vi "v3.21.v.vi"() -> ()   [LabVIEW 2018]
uses:
  <vilib>/DAQmx/read.llb/DAQmx Read (Analog 1D DBL NChan 1Samp).vi
  <extravilib>/ChannelInstances/High Speed Stream-c(a[.](c(dbl,dbl,dbl,dbl)),stamp,a[.](dbl),c(dbl,dbl,dbl,dbl,dbl,dbl,dbl))/_Read For Replicate.vi
  <extravilib>/ChannelInstances/High Speed Stream-c(a[.](c(dbl,dbl,dbl,dbl)),stamp,a[.](dbl),c(dbl,dbl,dbl,dbl,dbl,dbl,dbl))/Instantiate.vi
  <extravilib>/ChannelInstances/High Speed Stream-c(a[.](c(dbl,dbl,dbl,dbl)),stamp,a[.](dbl),c(dbl,dbl,dbl,dbl,dbl,dbl,dbl))/)Channel.vi
  <extravilib>/ChannelInstances/High Speed Stream-c(a[.](c(dbl,dbl,dbl,dbl)),stamp,a[.](dbl),c(dbl,dbl,dbl,dbl,dbl,dbl,dbl))/Abort Signal/Init Signal.vi
  <vilib>/Utility/file.llb/Write Delimited Spreadsheet (string).vi
  <vilib>/DAQmx/create/channels.llb/DAQmx Create Channel (AI-Temperature-Thermocouple).vi
  <vilib>/DAQmx/configure/timing.llb/DAQmx Timing (Sample Clock).vi
  <vilib>/DAQmx/miscellaneous.llb/DAQmx Fill In Error Info.vi
  <extravilib>/ChannelInstances/High Speed Stream-c(a[.](c(dbl,dbl,dbl,dbl)),stamp,a[.](dbl),c(dbl,dbl,dbl,dbl,dbl,dbl,dbl)).lvlib
panel:
  out "Current Time":timestamp
  out "DAQmx Data":T1
  out "Rig Temperatures":T2
  out "Flowrate Data":T3(array[cluster])
  out "UI Current Time":timestamp format="%<%X\n%x>T"
  out "DAQ Current Time":timestamp format="%<%X\n%x>T"
  in  "file path (dialog if empty)":path
  out "Enum":T4(ring)
  in  "Start Recording?":bool
  in  "Stop Recording?":bool
  in  "Flowrate Control":dbl
  out "Status":T5(ring)
  in  "OK Button":bool
  in  "DAQ Properties":cluster{"Sample Rate [Hz]":dbl}={"Sample Rate [Hz]"=1.0} {"Sample Rate [Hz]" min=0.1 max=10000.0 step=0.1}
  # "Line Data [ °C]"
  # "Rig Temperatures [ °C]"
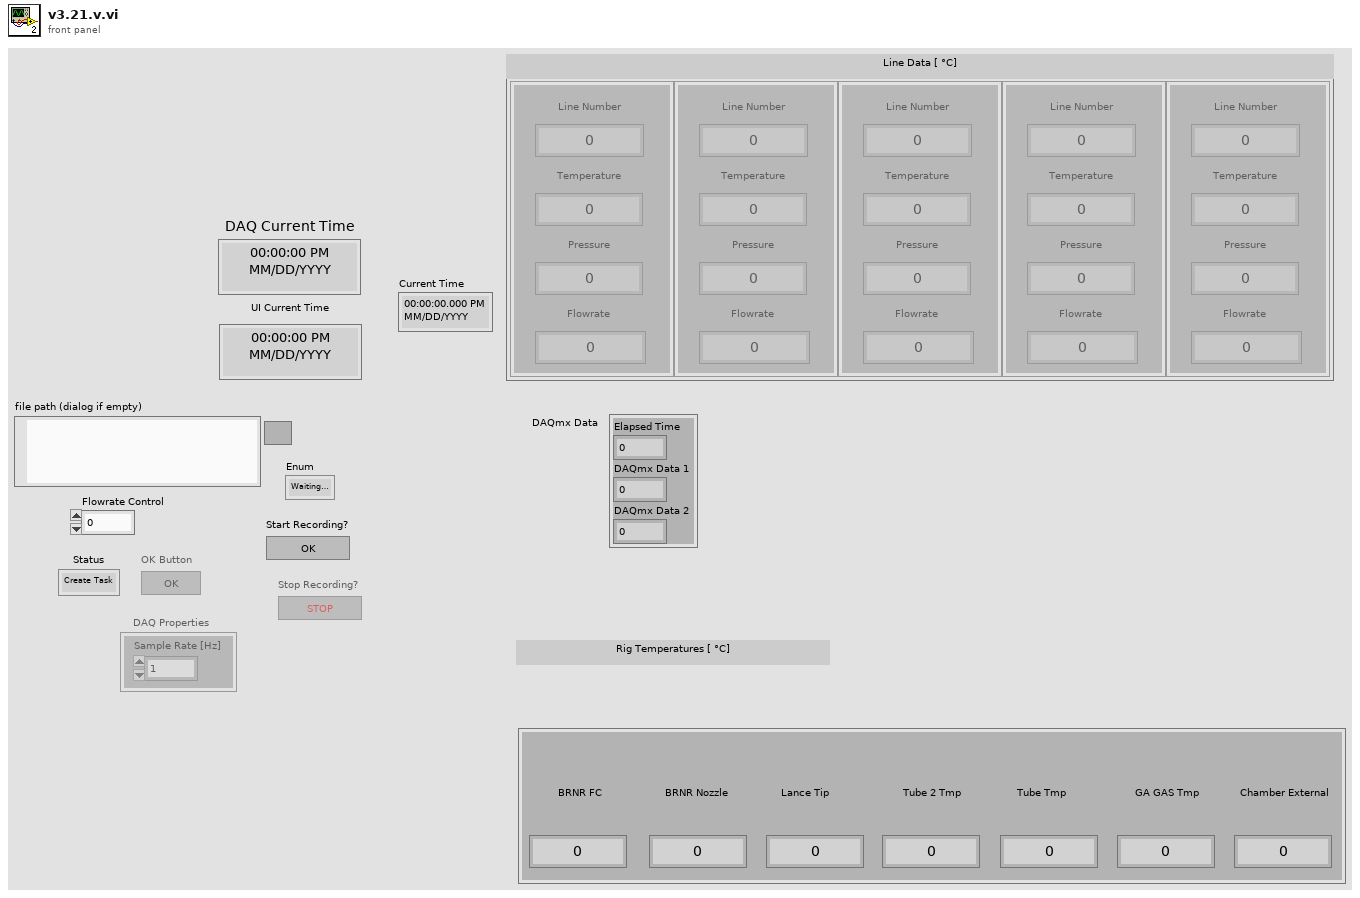
[diagram p1: front panel]
types:
  T1 = cluster{"Elapsed Time":dbl, "DAQmx Data 1":dbl, "DAQmx Data 2":dbl}
  T2 = cluster{"BRNR FC":dbl, "BRNR Nozzle":dbl, "Lance Tip":dbl, "Tube 2 Tmp":dbl, "Tube Tmp":dbl, "GA GAS Tmp":dbl, "Chamber External":dbl}
  T3 = cluster{"Line Number":dbl, "Temperature":dbl, "Pressure":dbl, "Flowrate":dbl}[]
  T4 = enum16{"Waiting to record", "Creating Spreadsheet", "Recording", "Finished Recording"}
  T5 = enum16{"Create Task", "Change Settings", "Check Settings", "Read Data", "End Task"}
  T6 = enum8{"Enabled", "Disabled", "Disabled and Grayed Out"}
  T7 = cluster{"Flowrate Data":cluster{"Line Number":dbl, "Temperature":dbl, "Pressure":dbl, "Flowrate":dbl}[], "Current Time":timestamp, "DAQmx Data":dbl[], "Rig Temperatures":cluster{"BRNR FC":dbl, "BRNR Nozzle":dbl, "Lance Tip":dbl, "Tube 2 Tmp":dbl, "Tube Tmp":dbl, "GA GAS Tmp":dbl, "Chamber External Temp":dbl}}
  T8 = cluster{"BRNR FC":dbl, "BRNR Nozzle":dbl, "Lance Tip":dbl, "Tube 2 Tmp":dbl, "Tube Tmp":dbl, "GA GAS Tmp":dbl, "Chamber External Temp":dbl}
  T9 = typedef "High Speed Stream-c(a[.](c(dbl,dbl,dbl,dbl)),stamp,a[.](dbl),c(dbl,dbl,dbl,dbl,dbl,dbl,dbl)).lvlib/)Channel.ctl" = refnum<queue>
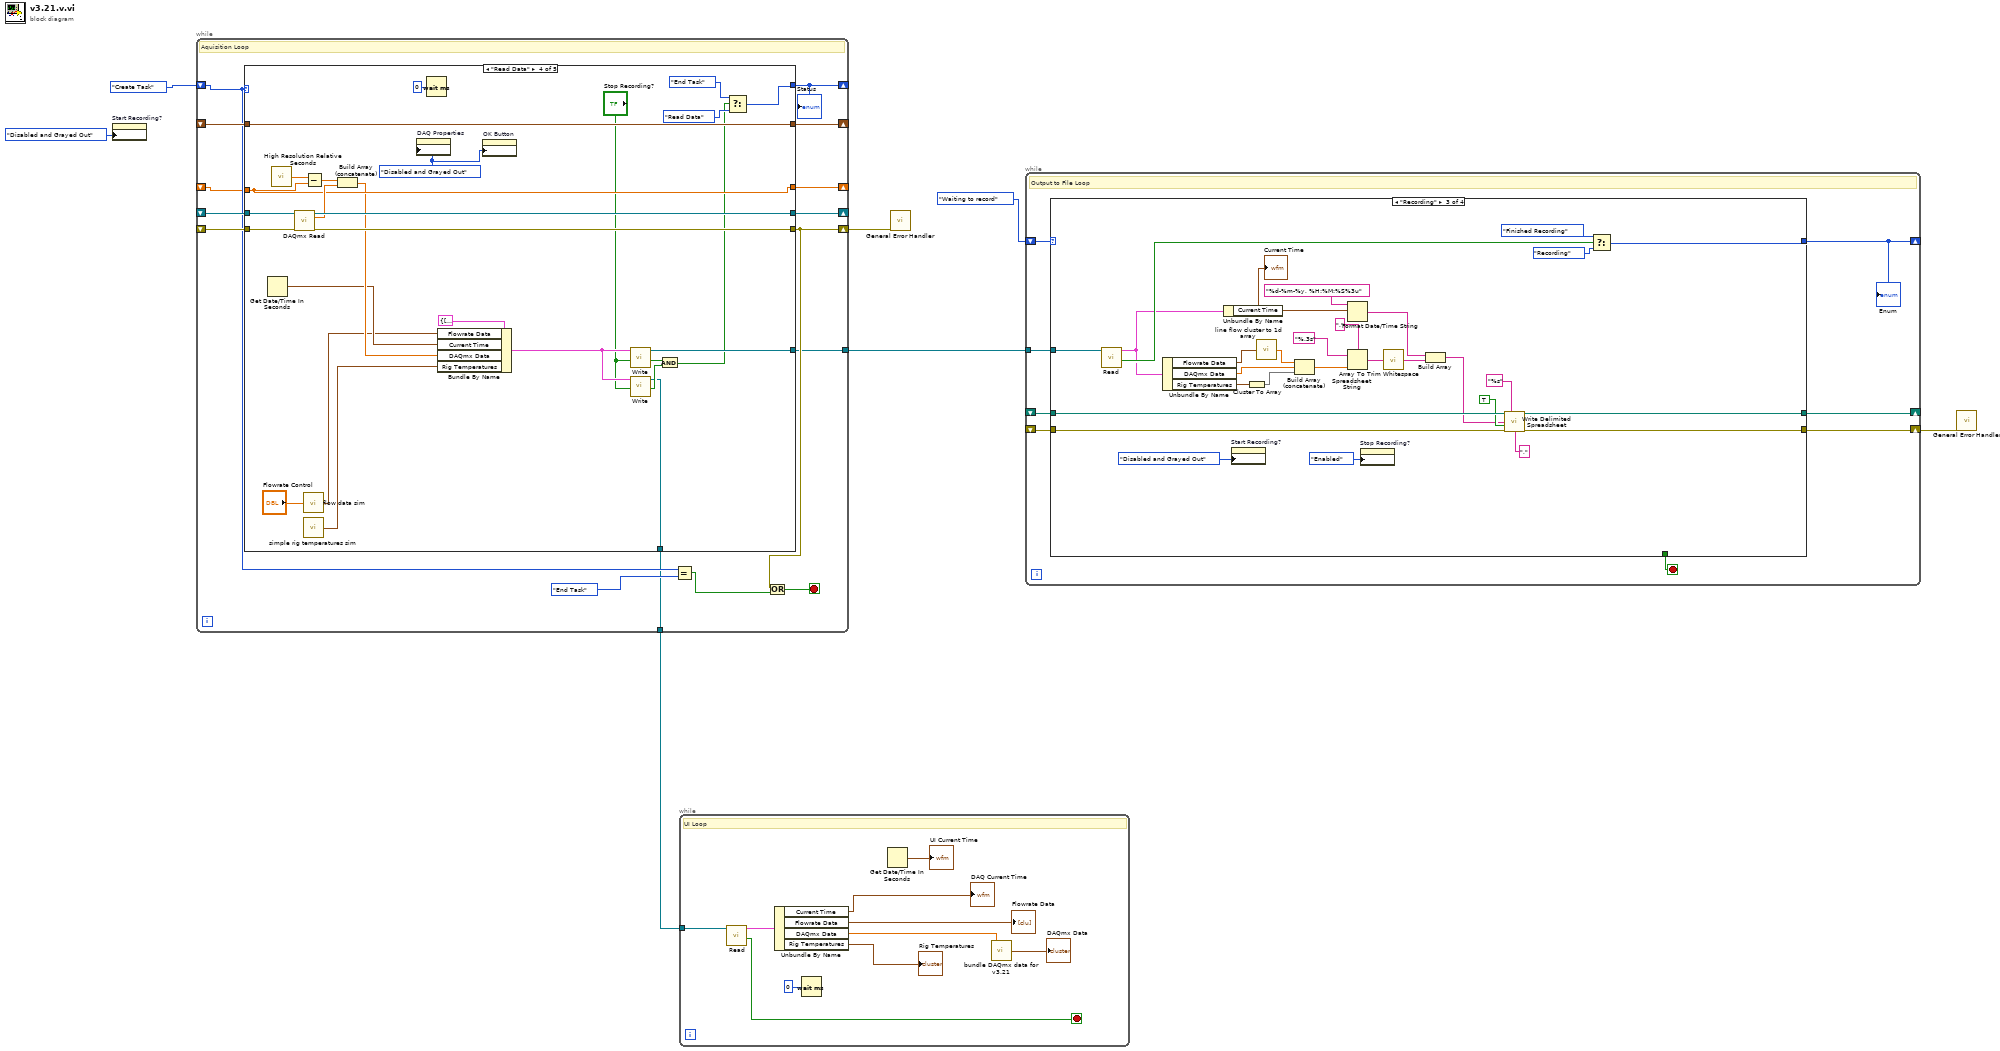
[diagram p0: block diagram]
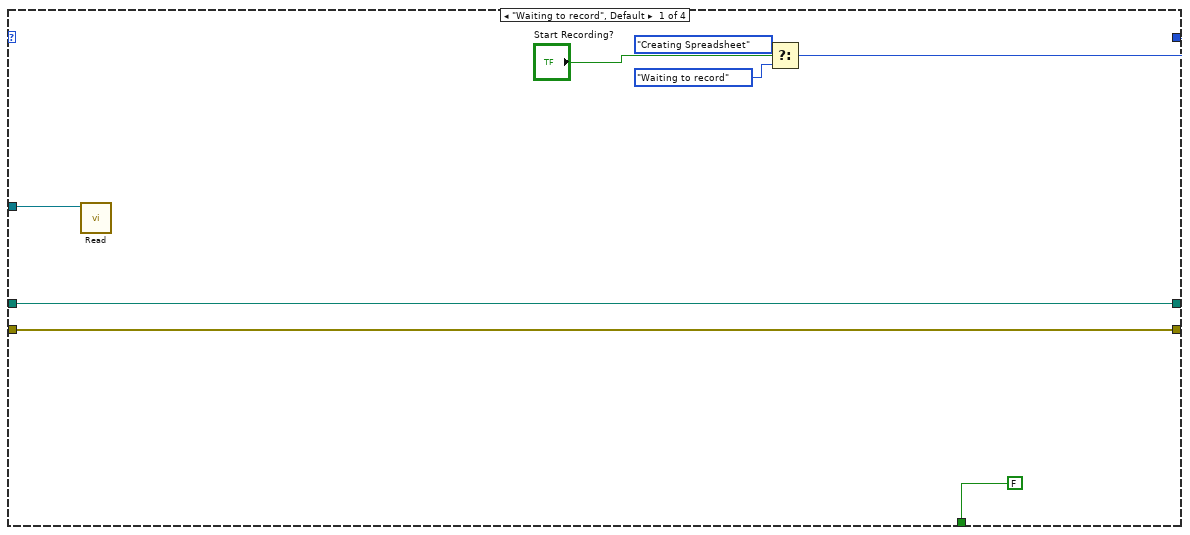
[diagram p2: hidden frame]
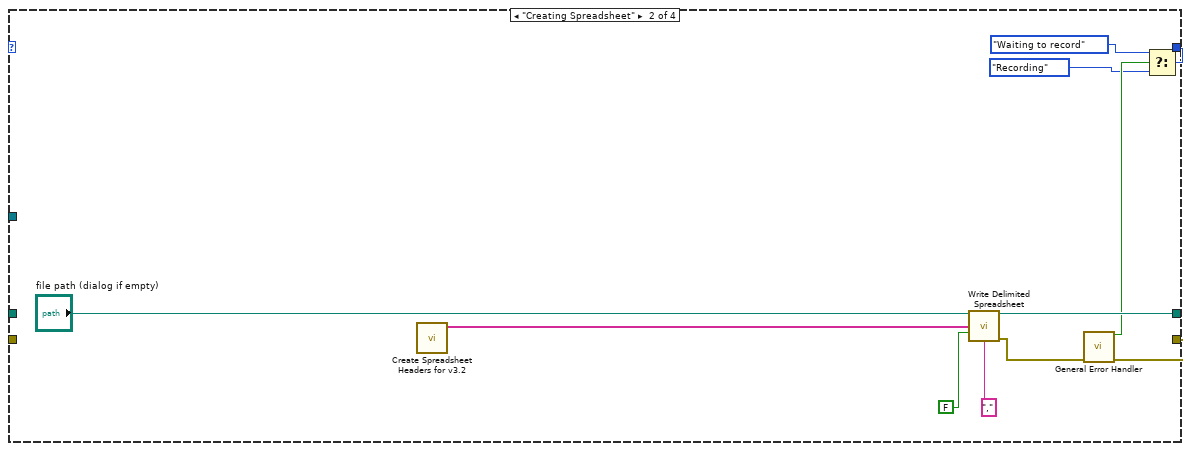
[diagram p3: hidden frame]
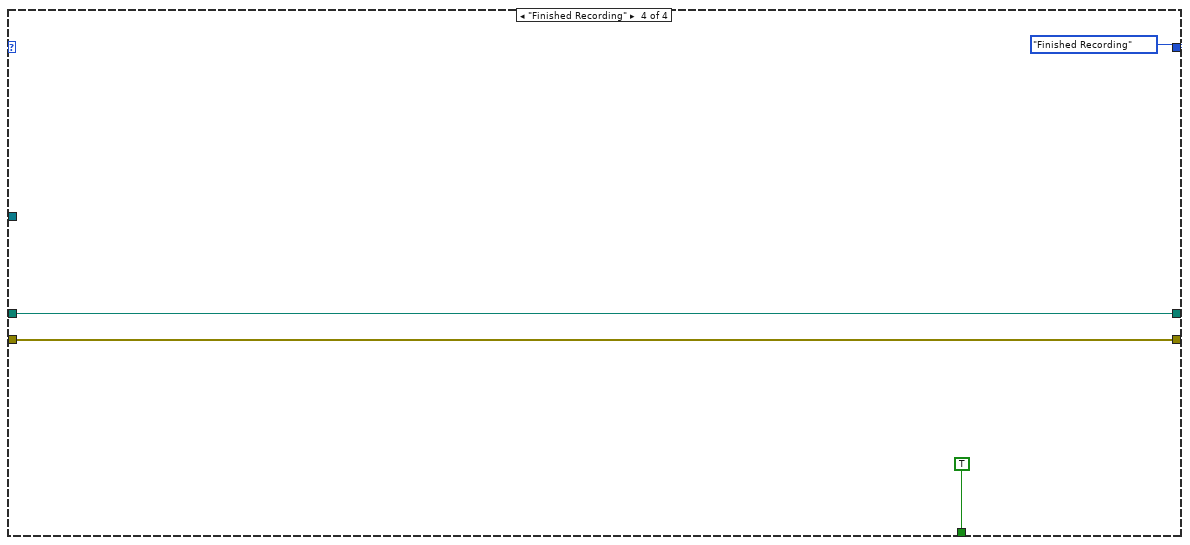
[diagram p4: hidden frame]
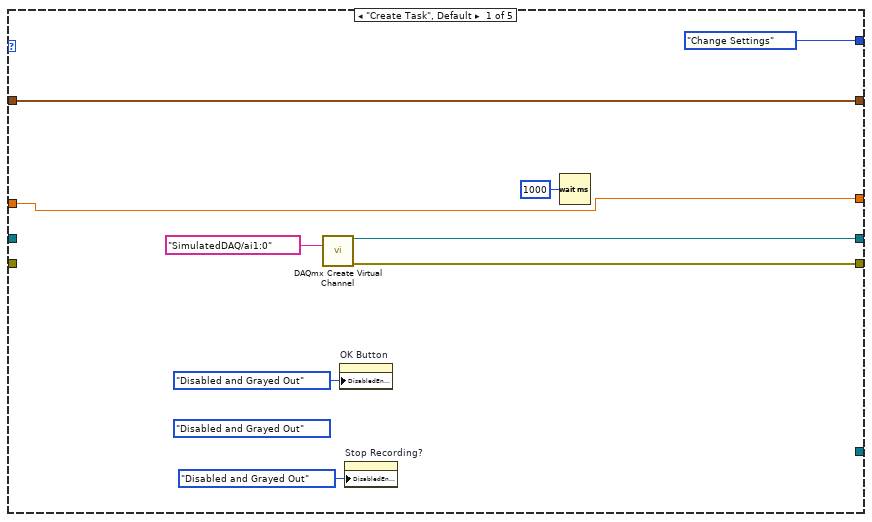
[diagram p5: hidden frame]
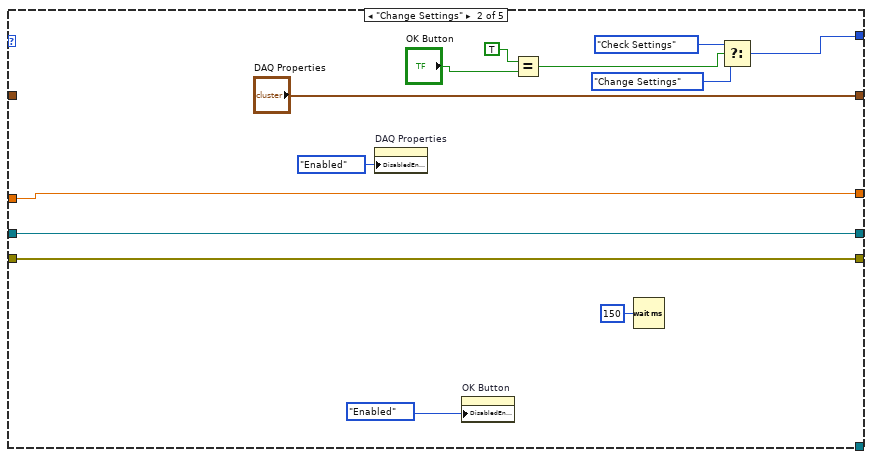
[diagram p6: hidden frame]
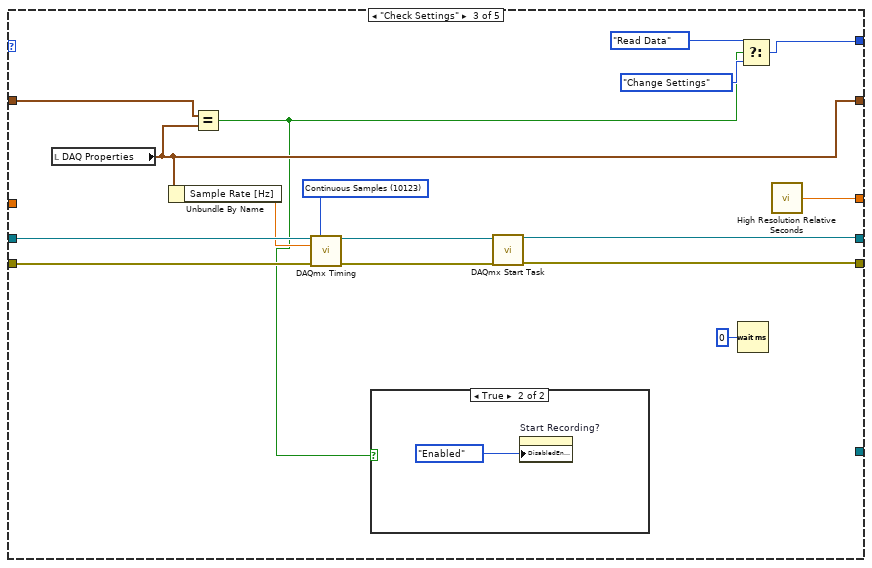
[diagram p7: hidden frame]
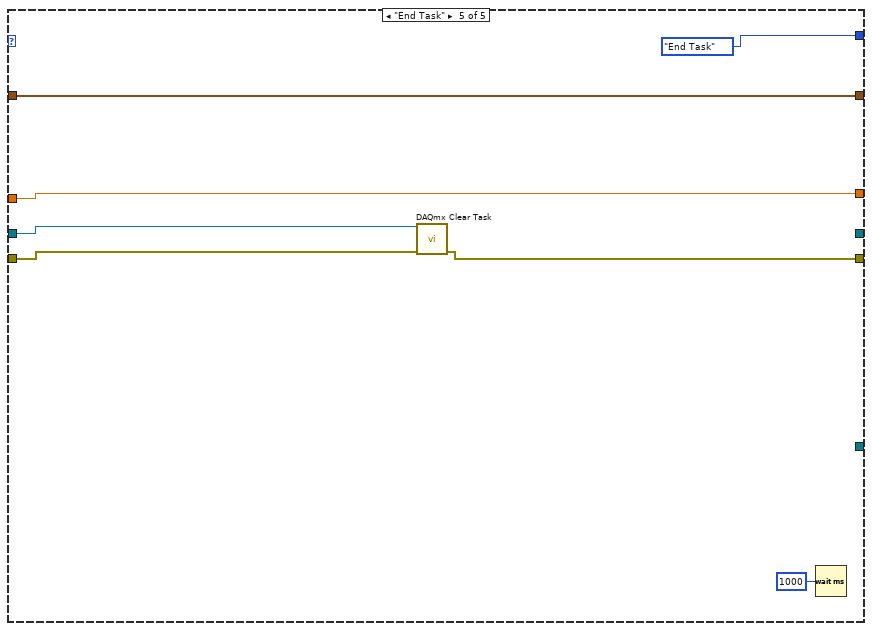
[diagram p9: hidden frame]
diagram:
  n1 = property on="Start Recording?" class="Bool"("DisabledEnum"=T6."Disabled and Grayed Out" ("Disabled")) -> ()  [unwired: 2 in, 2 out]
  n2 = while {
    shift-right: [w17] -> _
    shift-left: T5."Create Task" -> [w13]
    shift-right: [w22] -> _
    shift-left: _ -> [w20]
    shift-right: [w16] -> w3
    shift-left: _ -> [w19]
    shift-right: [w21] -> _
    shift-left: _ -> [w18]
    shift-right: [w12] -> _
    shift-left: _ -> [w11]
    tunnel: [w9] -> w5
    tunnel: [w8] -> w1
    stop <- w10 stop-if-true
    # "Aquisition Loop"
    n3 = case shown="\"Read Data\"" w13 {
      tunnel: [w31 w44 w49 w85 _] -> w22
      tunnel: [w30 w43 w48 w84 w95] -> w16
      tunnel: [T5."Change Settings" w37 w56 w82 T5."End Task"] -> w17
      tunnel: [w27 "DAQ Properties" w52 w86 w94] -> w21
      tunnel: w20 -> [_ w44 w55 w88 w92]
      tunnel: w19 -> [_ w43 w54 w87 w91]
      tunnel: w18 -> [w27 _ w60 w86 w94]
      tunnel: [w25 w34 w46 w76 w90] -> w12
      tunnel: w11 -> [w25 w34 _ w76 w90]
      tunnel: [_ _ _ w69 _] -> w9
      tunnel: [_ _ _ w62 _] -> w8
      frame "Create Task", Default {
        (unwired) T6."Disabled and Grayed Out" ("Disabled")
        n4 = call-poly <vilib>:"DAQmx Create Virtual Channel.vi"("physical channels"=tag "SimulatedDAQ/ai1:0") -> ("task out"=w31:refnum<k21>, "error out"=w30:errorcluster)  [unwired: 13 in]
        n5 = property on="OK Button" class="Bool"("DisabledEnum"=T6."Disabled and Grayed Out" ("Disabled")) -> ()  [unwired: 2 in, 2 out]
        n6 = property on="Stop Recording?" class="Bool"("DisabledEnum"=T6."Disabled and Grayed Out" ("Disabled")) -> ()  [unwired: 2 in, 2 out]
        n7 = Wait (ms)(milliseconds to wait=u32 1000) -> ()  [unwired: 1 out]
      }
      frame "Change Settings" {
        n8 = property on="DAQ Properties" class="Clust (strict)"("DisabledEnum"=T6."Enabled" ("Disabled")) -> ()  [unwired: 2 in, 2 out]
        n9 = property on="OK Button" class="Bool"("DisabledEnum"=T6."Enabled" ("Disabled")) -> ()  [unwired: 2 in, 2 out]
        n10 = Equal?(x=TRUE, y="OK Button") -> (x = y?=w39:bool)
        n11 = Wait (ms)(milliseconds to wait=u32 150) -> ()  [unwired: 1 out]
        n12 = Select(t=T5."Check Settings", s=w39, f=T5."Change Settings") -> (s? t:f=w37:T5)
      }
      frame "Check Settings" {
        w47 = 10123 items=["Finite Samples"=10178, "Continuous Samples"=10123, "Hardware Timed Single Point"=12522] ("sample mode")
        n13 = local read "DAQ Properties"() -> (w52:cluster{"Sample Rate [Hz]":dbl})
        n14 = Unbundle By Name(w52) -> ("Sample Rate [Hz]"=w53:dbl)
        n15 = Equal?(x=w60, y=w52) -> (x = y?=w45:bool)
        n16 = call-poly <vilib>:"DAQmx Timing.vi"("task/channels in"=w55, "sample mode"=w47, "rate"=w53, "error in"=w54) -> ("task out"=w51:refnum<k21>, "error out"=w50:errorcluster)  [unwired: 10 in]
        n17 = case shown="True" w45 {
          frame False {
          }
          frame True {
            n18 = property on="Start Recording?" class="Bool"("DisabledEnum"=T6."Enabled" ("Disabled")) -> ()  [unwired: 2 in, 2 out]
          }
        }
        n19 = call <vilib>:"DAQmx Start Task.vi"("task/channels in"=w51, "error in"=w50) -> ("task out"=w49:refnum<k21>, "error out"=w48:errorcluster)  [unwired: 12 in]
        n20 = Wait (ms)(milliseconds to wait=u32 0) -> ()  [unwired: 1 out]
        n21 = Select(t=T5."Read Data", s=w45, f=T5."Change Settings") -> (s? t:f=w56:T5)
        n22 = call <vilib>:"High Resolution Relative Seconds.vi"() -> ("relative seconds"=w46:dbl)
      }
      frame "Read Data" {
        w68 = T6."Disabled and Grayed Out" ("Disabled")
        n23 = Get Date/Time In Seconds() -> (seconds since 1Jan1904=w72:timestamp)
        n24 = call <vilib>:"High Resolution Relative Seconds.vi"() -> ("relative seconds"=w79:dbl)
        n25 = call-poly <vilib>:"DAQmx Read.vi"("task/channels in"=w88, "error in"=w87) -> ("task out"=w85:refnum<k21>, "data"=w78:dbl[], "error out"=w84:errorcluster)  [unwired: 11 in]
        n26 = call "simple rig temperatures sim.vi"() -> ("Rig Temperatures"=w70:T8)
        n27 = call "flow data sim.vi"("Boondoggle Input"="Flowrate Control") -> ("Flowrate Data"=w71:T3)
        n28 = Subtract(x=w79, y=w76) -> (x-y=w77:dbl)
        n29 = Build Array (concatenate)(w77, w78) -> (w73:dbl[])
        n30 = property on="DAQ Properties" class="Clust (strict)"("DisabledEnum"=w68) -> ()  [unwired: 2 in, 2 out]
        n31 = Wait (ms)(milliseconds to wait=u32 0) -> ()  [unwired: 1 out]
        n32 = Bundle By Name(cluster=T7 {"Flowrate Data"=[{"Line Number"=1.0, "Temperature"=17.480721541683437, "Pressure"=24.0, "Flowrate"=0.0}, {"Line Number"=2.0, "Temperature"=21.850901927104296, "Pressure"=30.0, "Flowrate"=0.0}, {"Line Number"=3.0, "Temperature"=26.221082312525155, "Pressure"=36.0, "Flowrate"=0.0}, {"Line Number"=4.0, "Temperature"=30.591262697946018, "Pressure"=42.00000000000001, "Flowrate"=0.0}, {"Line Number"=5.0, "Temperature"=34.96144308336687, "Pressure"=48.0, "Flowrate"=0.0}], "Current Time"=timestamp(0 s since 1904-01-01), "DAQmx Data"=[], "Rig Temperatures"={"BRNR FC"=0.0, "BRNR Nozzle"=0.0, "Lance Tip"=0.0, "Tube 2 Tmp"=0.0, "Tube Tmp"=0.0, "GA GAS Tmp"=0.0, "Chamber External Temp"=0.0}}, "Flowrate Data"=w71, "Current Time"=w72, "DAQmx Data"=w73, "Rig Temperatures"=w70) -> (w67:T7)
        n33 = property on="OK Button" class="Bool"("DisabledEnum"=w68) -> ()  [unwired: 2 in, 2 out]
        n34 = call <extravilib>:"Write.vi"("last element? (F)"="Stop Recording?", "element"=w67) -> ("done?"=w65:bool, "channel"=w69:T9)  [unwired: 7 in, 1 out]
        n35 = call <extravilib>:"Write.vi"("last element? (F)"="Stop Recording?", "element"=w67) -> ("done?"=w64:bool, "channel"=w62:T9)  [unwired: 7 in, 1 out]
        n36 = And(x=w65, y=w64) -> (x .and. y?=w63:bool)
        n37 = Select(t=T5."End Task", s=w63, f=T5."Read Data") -> (s? t:f=w82:T5)
      }
      frame "End Task" {
        n38 = call <vilib>:"DAQmx Clear Task.vi"("task in"=w92, "error in"=w91) -> ("error out"=w95:errorcluster)  [unwired: 13 in]
        n39 = Wait (ms)(milliseconds to wait=u32 1000) -> ()  [unwired: 1 out]
      }
    }
    "Status" <- w17
    n40 = Equal?(x=w13, y=T5."End Task") -> (x = y?=w14:bool)
    n41 = Or(x=w16, y=w14) -> (x .or. y?=w10:bool)
  }
  n42 = while {
    tunnel: w1 -> [w105]
    stop <- w104 stop-if-true
    # "UI Loop"
    n43 = call <extravilib>:"Read.vi"("channel"=w105) -> ("done?"=w104:bool, "element"=w102:T7)  [unwired: 6 in, 3 out]
    n44 = Unbundle By Name(w102) -> ("Current Time"=→"DAQ Current Time":timestamp, "Flowrate Data"=→"Flowrate Data":T3, "DAQmx Data"=w98:dbl[], "Rig Temperatures"=→"Rig Temperatures":T8)
    n45 = Wait (ms)(milliseconds to wait=u32 0) -> ()  [unwired: 1 out]
    n46 = Get Date/Time In Seconds() -> (seconds since 1Jan1904=→"UI Current Time":timestamp)
    n47 = call "bundle DAQmx data for v3.21 .vi"("DAQmx Data"=w98) -> ("DAQmx Data"=→"DAQmx Data":T1)
  }
  n48 = call <vilib>:"General Error Handler.vi"("error in (no error)"=w3) -> ()  [unwired: 10 in, 5 out]
  n49 = while {
    shift-right: [w113] -> _
    shift-left: T4."Waiting to record" -> [w112]
    tunnel: w5 -> [w110]
    shift-right: [w108] -> _
    shift-left: _ -> [w109]
    shift-right: [w107] -> w4
    shift-left: _ -> [w106]
    stop <- w111 stop-if-true
    # "Output to File Loop"
    n50 = case shown="\"Recording\"" w112 {
      tunnel: [w118 w124 w160 T4."Finished Recording"] -> w113
      tunnel: [FALSE _ _ TRUE] -> w111
      tunnel: w110 -> [w114 _ w156 _]
      tunnel: w109 -> [w116 _ w153 w163]
      tunnel: [w116 w132 w154 w163] -> w108
      tunnel: [w115 w126 w133 w162] -> w107
      tunnel: w106 -> [w115 _ w144 w162]
      frame "Waiting to record", Default {
        n51 = call <extravilib>:"Read.vi"("channel"=w114) -> ()  [unwired: 6 in, 5 out]
        n52 = Select(t=T4."Creating Spreadsheet", s="Start Recording?", f=T4."Waiting to record") -> (s? t:f=w118:T4)
      }
      frame "Creating Spreadsheet" {
        n53 = call "Create Spreadsheet Headers for v3.2.vi"() -> ("Array"=w131:string[])  [unwired: 11 in]
        n54 = call-poly <vilib>:"Write Delimited Spreadsheet.vi"("file path (dialog if empty)"="file path (dialog if empty)", "1D data"=w131, "append to file? (new file:F)"=FALSE, "delimiter (\\t)"="," ("delimiter (\\t)")) -> ("new file path (Not A Path if cancelled)"=w132:path, "error out"=w127:errorcluster)  [unwired: 10 in]
        n55 = call <vilib>:"General Error Handler.vi"("error in (no error)"=w127) -> ("error?"=w125:bool, "error out"=w126:errorcluster)  [unwired: 10 in, 3 out]
        n56 = Select(t=T4."Waiting to record", s=w125, f=T4."Recording") -> (s? t:f=w124:T4)
      }
      frame "Recording" {
        n57 = call <extravilib>:"Read.vi"("channel"=w156) -> ("done?"=w155:bool, "element"=w150:T7)  [unwired: 6 in, 3 out]
        n58 = Unbundle By Name(w150) -> ("Flowrate Data"=w151:T3, "DAQmx Data"=w148:dbl[], "Rig Temperatures"=w157:T8)
        n59 = Unbundle By Name(w150) -> ("Current Time"=w135:timestamp)
        "Current Time" <- w135
        n60 = property on="Start Recording?" class="Bool"("DisabledEnum"=T6."Disabled and Grayed Out" ("Disabled")) -> ()  [unwired: 2 in, 2 out]
        n61 = Cluster To Array(cluster=w157) -> (array=w149:dbl[])
        n62 = call "line flow cluster to 1d array.vi"("Flowrate Data"=w151) -> ("Array"=w147:dbl[])
        n63 = Build Array (concatenate)(w147, w148, w149) -> (w146:dbl[])
        n64 = Format Date/Time String(time format string (%c)="%d-%m-%y, %H:%M:%S%3u", seconds (now)=w135) -> (date/time string=w137:string)  [unwired: 1 in]
        n65 = Array To Spreadsheet String(delimiter (Tab)=",", array=w146, 3:"%.3s" ("format string")) -> (spreadsheet string=w141:string)
        n66 = property on="Stop Recording?" class="Bool"("DisabledEnum"=T6."Enabled" ("Disabled")) -> ()  [unwired: 2 in, 2 out]
        n67 = call <vilib>:"Trim Whitespace.vi"("string"=w141) -> ("trimmed string"=w140:string)  [unwired: 1 in]
        n68 = Build Array(w137, w140) -> (w142:string[])
        n69 = call-poly <vilib>:"Write Delimited Spreadsheet.vi"("file path (dialog if empty)"=w153, "format (%s)"="%s", "1D data"=w142, "append to file? (new file:F)"=TRUE, "error in (no error)"=w144, "delimiter (\\t)"="," ("delimiter (\\t)")) -> ("new file path (Not A Path if cancelled)"=w154:path, "error out"=w133:errorcluster)  [unwired: 8 in]
        n70 = Select(t=T4."Finished Recording", s=w155, f=T4."Recording") -> (s? t:f=w160:T4)
      }
      frame "Finished Recording" {
      }
    }
    "Enum" <- w113
  }
  n71 = call <vilib>:"General Error Handler.vi"("error in (no error)"=w4) -> ()  [unwired: 10 in, 5 out]
